vi "Close SQL Connection.vi"(8 "error in (no error)":errorcluster, 11 "SQLObject in":refnum<class "SQLObject.lvclass">) -> (0 "error out":errorcluster, 3 "SQLObject out":refnum<class "SQLObject.lvclass">)   [LabVIEW 2021, in "SQLObject.lvclass"]
uses:
  SQLObject.lvclass
  SQLObject.lvclass/SQLObject.ctl
  <vilib>/drjdpowell/SQLite Library/SQL Connection/Connection.lvclass
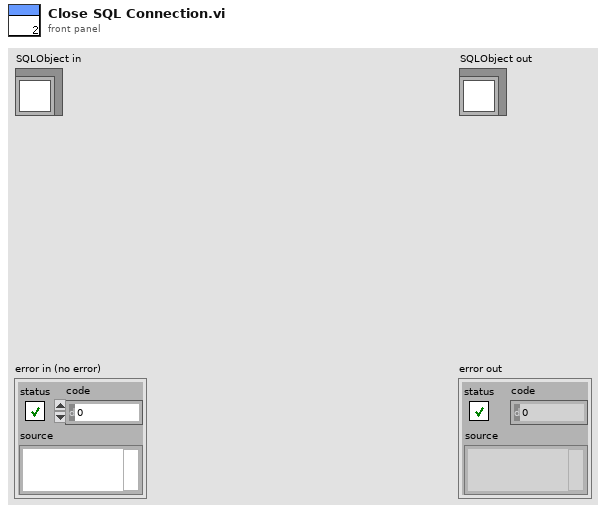
[diagram p1: front panel]
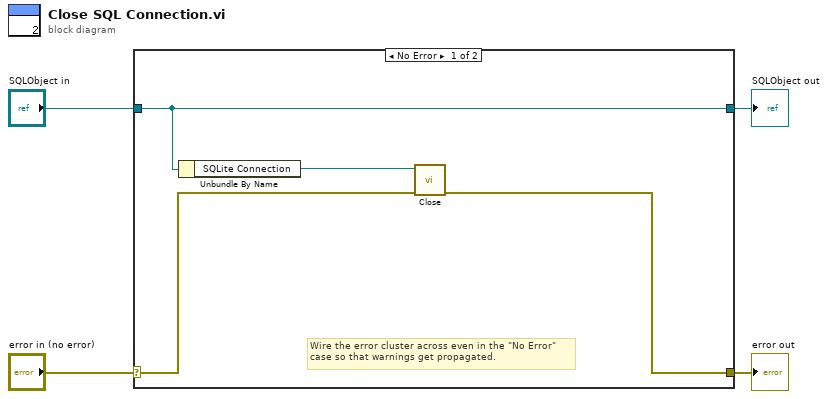
[diagram p0: block diagram]
diagram:
  n1 = case shown="No Error" "error in (no error)" {
    selector: "error in (no error)" -> [w6 w10]
    tunnel: [w5 w10] -> w3
    tunnel: [w8 w9] -> w1
    tunnel: "SQLObject in" -> [w8 w9]
    frame No Error {
      # "Wire the error cluster across even in the \"No Error\"\ncase so that warnings get propagated."
      n2 = Unbundle By Name(w8) -> ("SQLite Connection"=w7:refnum<class "Connection.lvclass">)
      n3 = call-dynamic "Close.vi"("error in (no error)"=w6, "SQLite Connection in"=w7) -> ("error out"=w5:errorcluster)  [unwired: 9 in]
    }
    frame Error {
    }
  }
  "error out" <- w3
  "SQLObject out" <- w1
